vi "RT Main 9039.vi"() -> ()   [LabVIEW 2018]
doc: "This template is for the Queued Message Handler design pattern.\n\nThe Event Handling Loop generates messages based on user interface actions.\n\nThe Message Handling Loop processes messages generated by the Event Handling Loop, or by other messages. The messages are string values, so new messages can be added easily to the Message Cases case structure in the Message Handling Loop. Each message cluster can also provide an optional value for Message Data, which is a variant that can be converted to whatever message-specific data is required."
uses:
  controls/FPGA State.ctl
  controls/Fill Valves.ctl
  controls/VENT SYSTEM.ctl
  controls/LNG PUGE.ctl
  controls/LOX PURGE.ctl
  Globals/Global - All RT Loop Stop.vi
  Globals/Global - Configuration Options.vi
  COMET  Extra Programs/Globals/Global - Monitoring Variables.vi
  <vilib>/rvi/errors/niLvFpgaAdjustHostInterfaceError.vi
  Globals/Global - RT Stream Connections.vi
  <vilib>/FPGAPlugInAG/Dynamic/niLvFpga_Close_Dynamic.vi
  <vilib>/rvi/interface/nirviReadWriteControl/nirviReadWriteControl.xnode
  controls/FPGA VI Reference.ctl
  <vilib>/rvi/interface/nirviCloseFPGA/nirviCloseFPGA.xnode
  support/Message Queue/Message Queue.lvlib
  NiFpgaLv.dll
  <vilib>/rvi/interface/Simulation/niFpgaSimulationCallBeginRW.vi
  <vilib>/nisyscfg/nisyscfg.lvlib
panel:
  out "data 2":enum16{"Standard", "Grill", "ROFI"}(ring)
  out "MOD 2 error":bool
  out "Input Error":bool
  out "Watchdog Timed Out?":bool
  out "Current FPGA State":enum16{"Safe State", "Manual", "Control"}(ring)
  out "data":T1
  out "MOD 6 Error":bool
  out "LNG_BV":bool
  out "LOX_BV":bool
  out "dup error to report":errorcluster
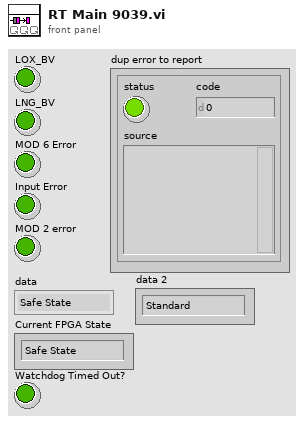
[diagram p1: front panel]
types:
  T1 = typedef "FPGA State.ctl" = enum16{"Safe State", "Manual", "Control"}
  T2 = typedef "Acquisition and Logging Configuration.ctl" = cluster{"Samples per Read 9237":i32, "Number of Reads to Save":i32, "Data File Name 9222_9039_EXP":string, "TDMS Properties 9222":T3[], "Number of Channels 9237_9049_MAIN":i32, "Trigger - RMS Value":dbl, "Trigger - Channel":i32, "Trigger - Time (Minute)":i32, "Data Rate 9237":T4, "Number of Channels 9222_9039_EXP":i32, "Samples per Read 9222":i32, "Data Rate 9222":i32, "Channel Names 9222_9039_EXP":string[], "TDMS Properties 9237":T3[], "Data File Name 9237_9049":string, "Excitation Voltage":T5, "Data File Name 9222_9049_MAIN":string, "Number of Channels 9222_9049_MAIN":i32, "Channel Names 9222_9049_MAIN":string[], "Data File Name 9237_9039":string, "Channel Names 9237_9039_EXP":string[], "Channel Names 9237_9049_MAIN":string[], "Number of Channels 9237_9039_EXP":i32}
  T3 = typedef "TDMS Properties.ctl" = cluster{"Name":string, "Value":string}
  T4 = typedef "nicrio_cRIO-9237_DataRatesRing.ctl" = u8
  T5 = typedef "nicrio_cRIO-9237_ExcitationVoltageRing.ctl" = u8
  T6 = typedef "EXPANSION FPGA VI Reference.ctl" = refnum<k20>
  T7 = typedef "FPGA VI Reference.ctl" = refnum<k20>
  T8 = typedef "Message Queue.lvlib/All Real-Time Message Queues Multi Queues.ctl" = cluster{"Message Handler":refnum<queue>, "Acquisition and Logging 9237":refnum<queue>, "Emergeny Stop for DCs":refnum<queue>, "LNG DC Commands":refnum<queue>, "LOX DC Commands":refnum<queue>, "Acquisition and Logging 9222":refnum<queue>, "Acquisition and Logging 9222_MAIN":refnum<queue>, "AUTO P&D":refnum<queue>, "Pressure Control":refnum<queue>}
  T9 = typedef "VENT SYSTEM.ctl" = cluster{"LNG_BFV":bool, "LOX_BFV":bool, "NGV_GV":bool}
  T10 = typedef "LNG PUGE.ctl" = cluster{"LNG_USP":bool, "LNG_DSP":bool}
  T11 = typedef "LOX PURGE.ctl" = cluster{"LOX_USP":bool, "LOX_DSP":bool}
  T12 = typedef "All FPGA Configuration Values.ctl" = cluster{"FPGA State":T1, "Manual Values":T13, "Fill Valves":T14, "LNG Purge System":T10, "LOX Purge System":T11, "DECOUPLERS":T15, "VENT SYSTEM":T9}
  T13 = typedef "Raw Values.ctl" = cluster{"LNG_VCV_POS":i16, " LOX_VCV_POS":i16, "LNG_VCV_CLOSE":bool, "LOX_VCV_CLOSE":bool, "LNG_BV_OPEN":bool, "LNG_BV_CLOSE":bool, "LOX_BV_OPEN":bool, "LOX_BV_CLOSE":bool, "LNG_BFV_OPEN":bool, "LNG_BFV_CLOSE":bool, "LOX_BFV_OPEN":bool, "LOX_BFV_CLOSE":bool}
  T14 = typedef "Fill Valves.ctl" = cluster{"LOX_BV":bool, "LNG_BV":bool, "LNG_VCV_CTL":sgl, "LOX_VCV_CTL":sgl}
  T15 = typedef "DECOUPLERS.ctl" = cluster{"LNG_DC":bool, "LOX_DC":bool, "NGV_DC":bool}
  T16 = cluster{"LOX_BV":bool, "LNG_BV":bool, "LNG_VCV_CTL":sgl, "LOX_VCV_CTL":sgl}
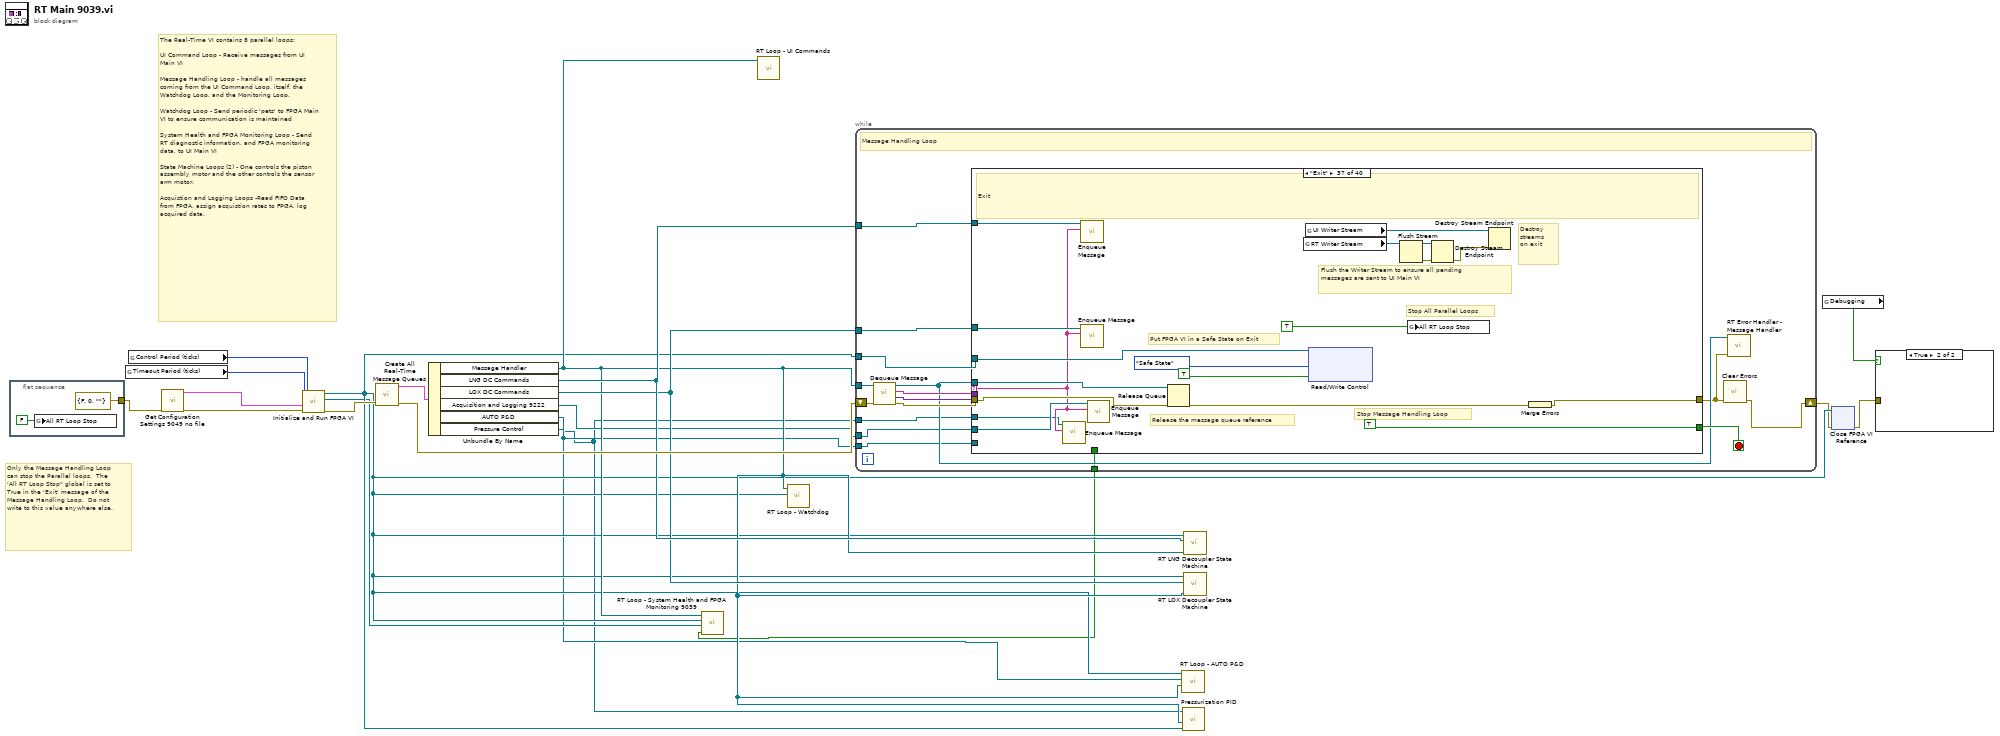
[diagram p0: block diagram]
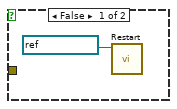
[diagram p2: hidden frame]
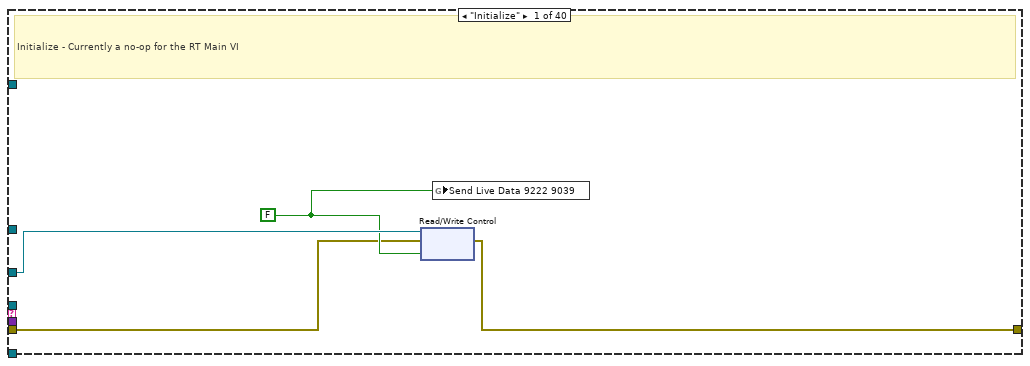
[diagram p3: hidden frame]
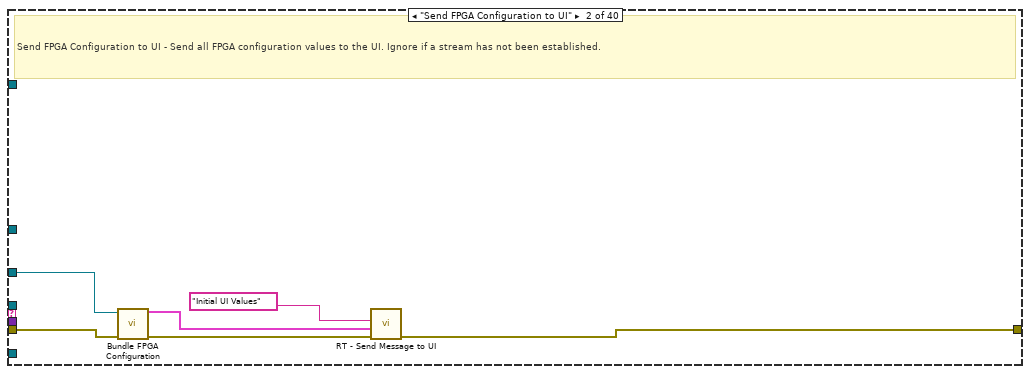
[diagram p4: hidden frame]
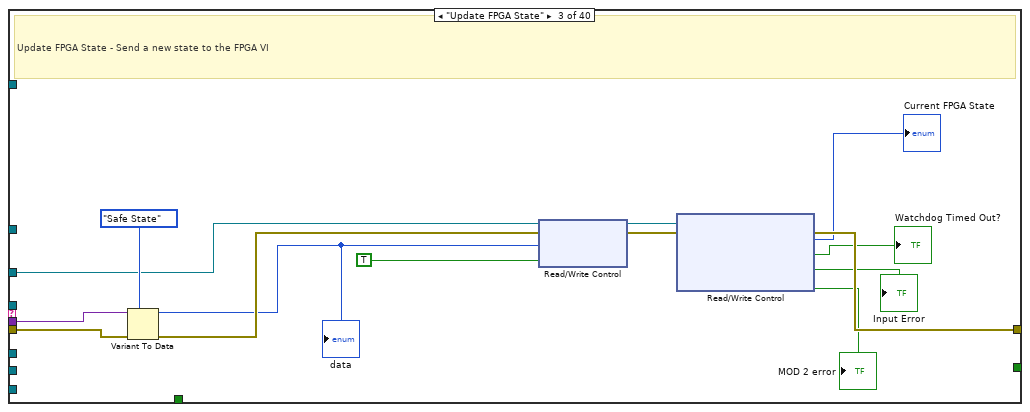
[diagram p5: hidden frame]
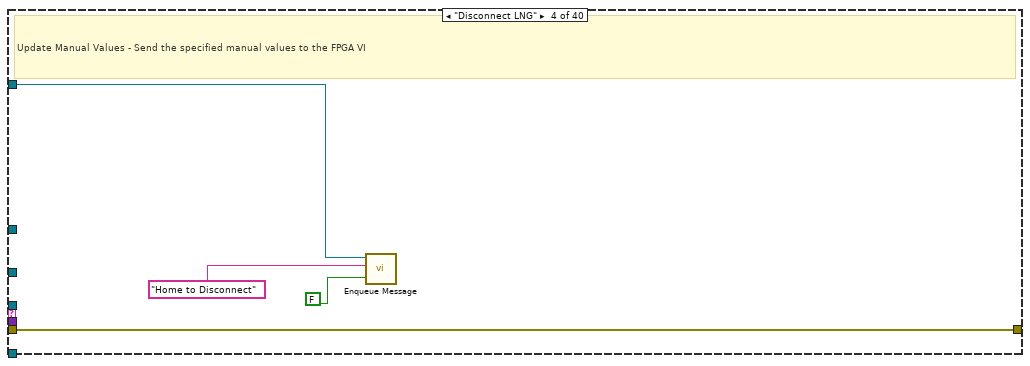
[diagram p6: hidden frame]
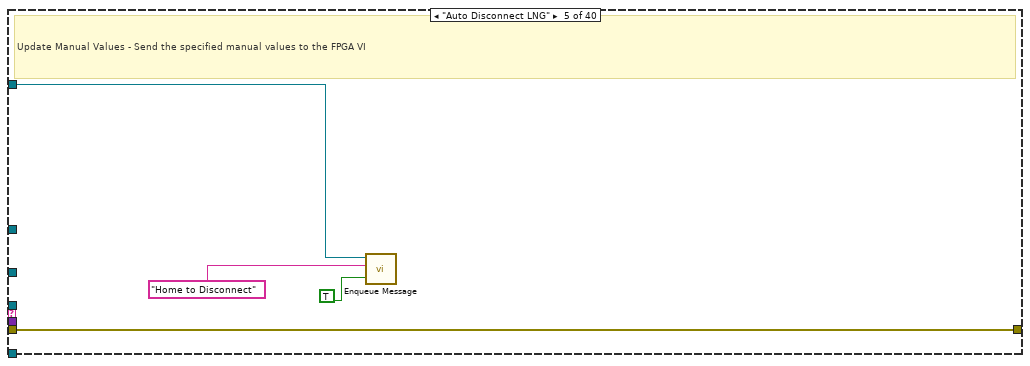
[diagram p7: hidden frame]
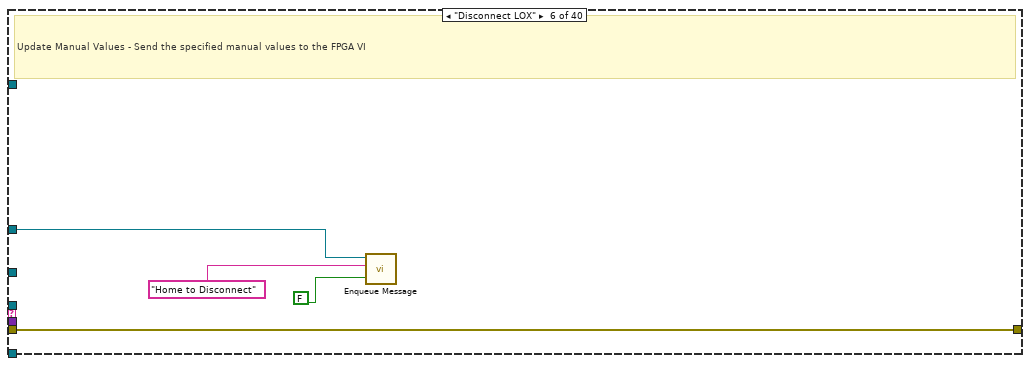
[diagram p8: hidden frame]
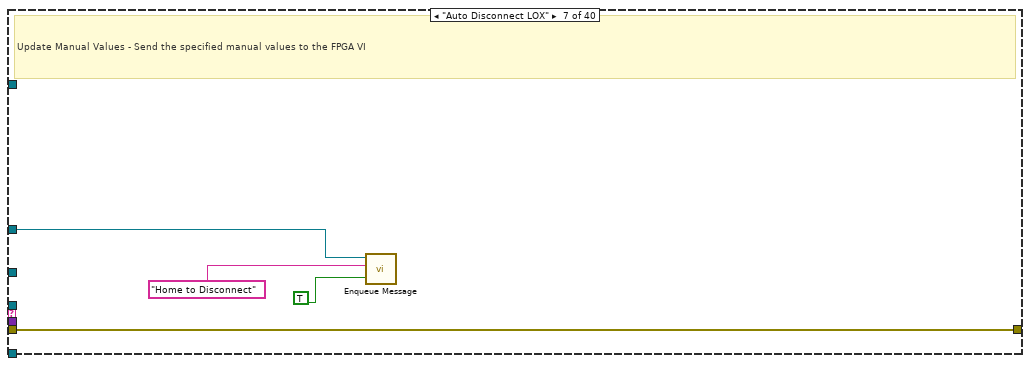
[diagram p9: hidden frame]
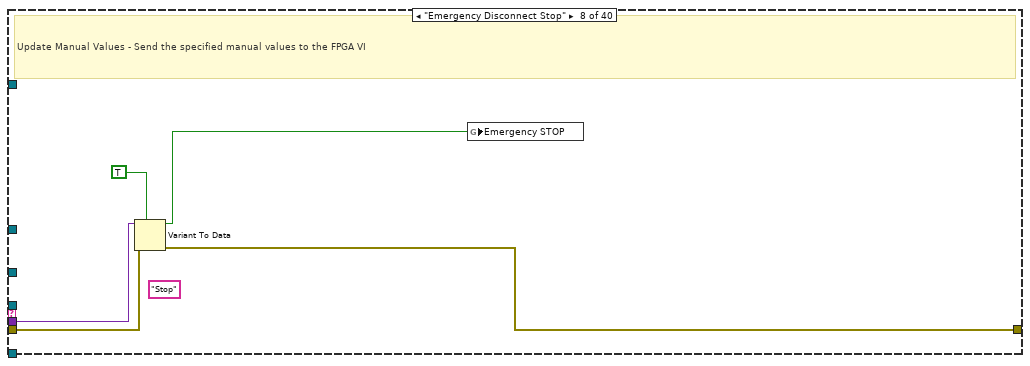
[diagram p10: hidden frame]
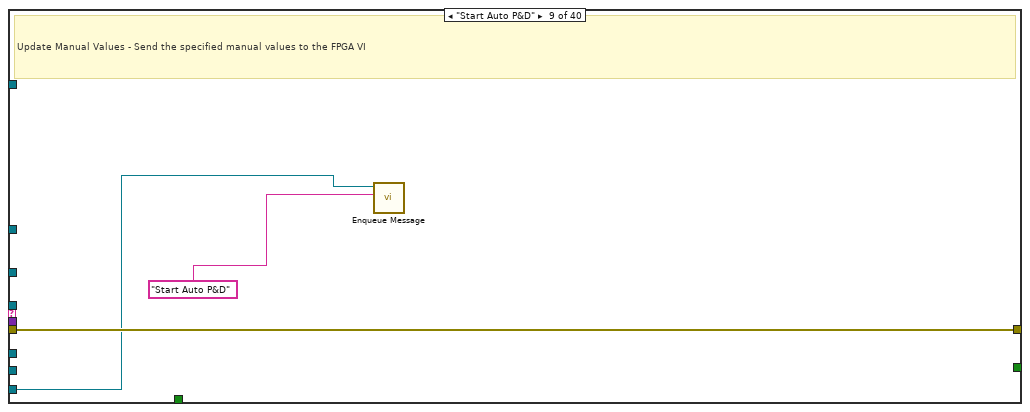
[diagram p11: hidden frame]
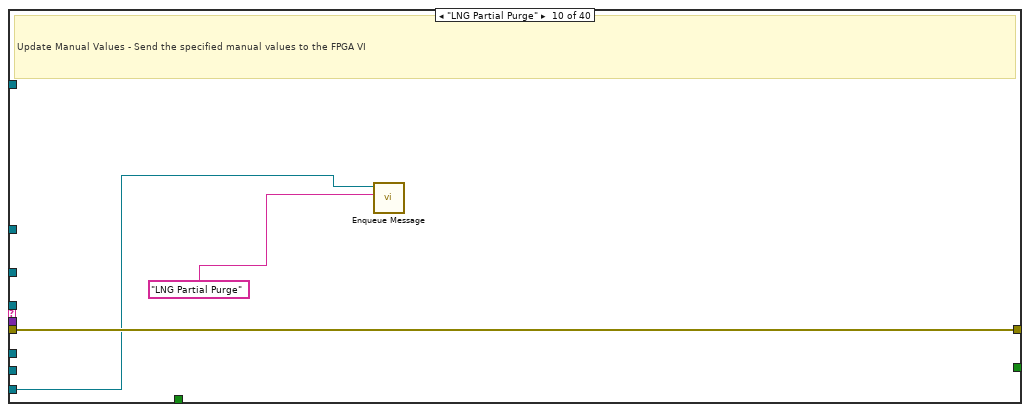
[diagram p12: hidden frame]
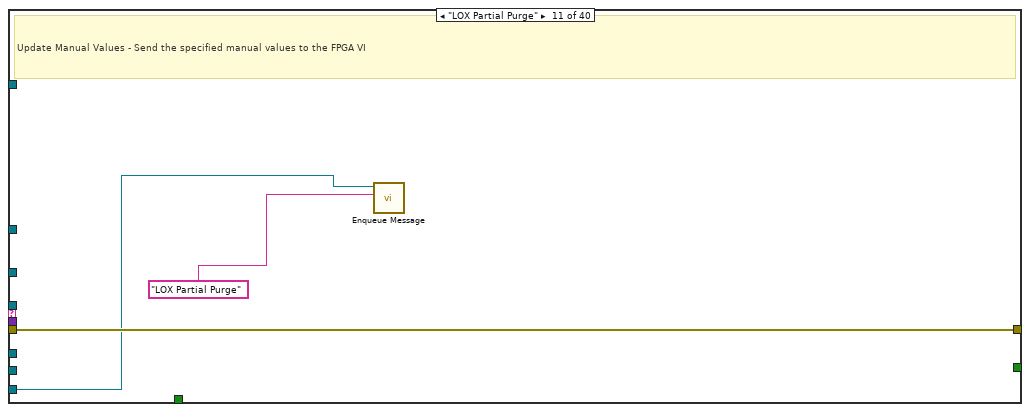
[diagram p13: hidden frame]
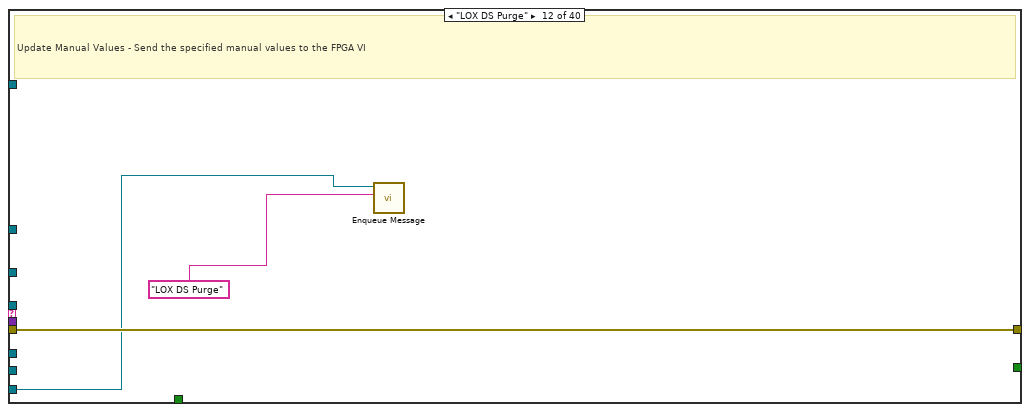
[diagram p14: hidden frame]
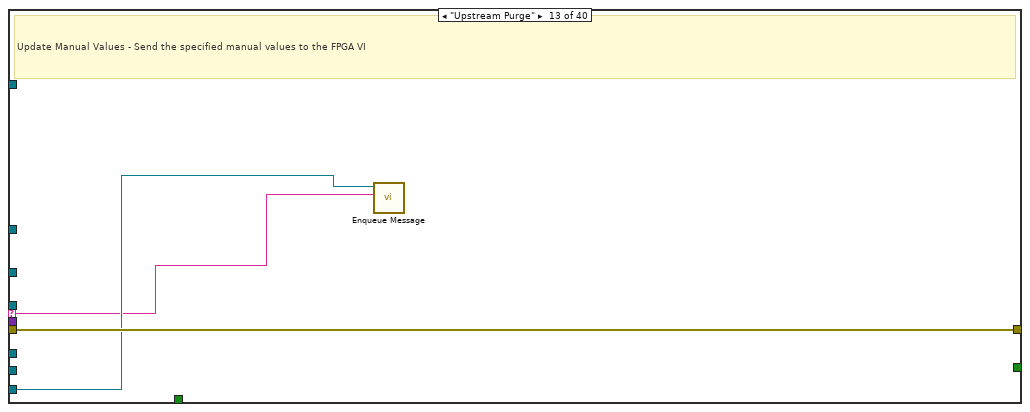
[diagram p15: hidden frame]
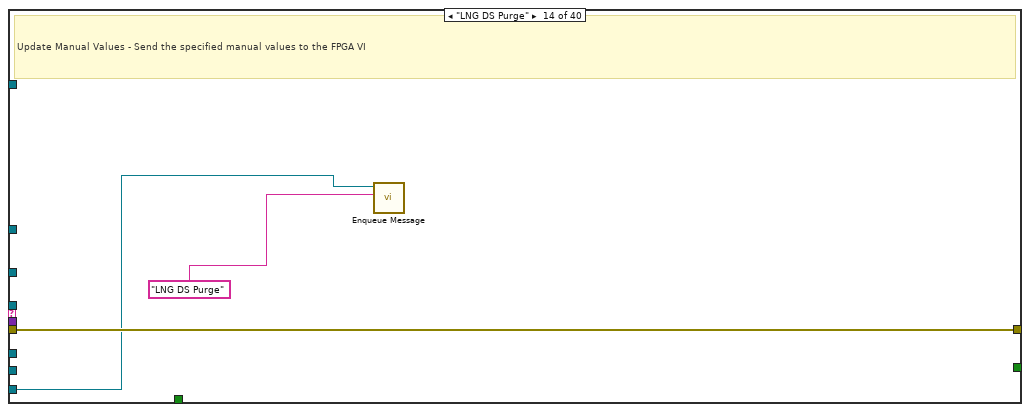
[diagram p16: hidden frame]
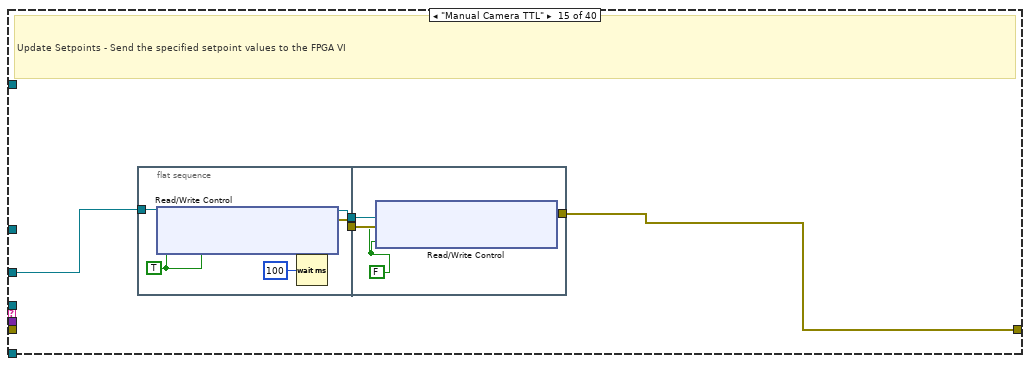
[diagram p17: hidden frame]
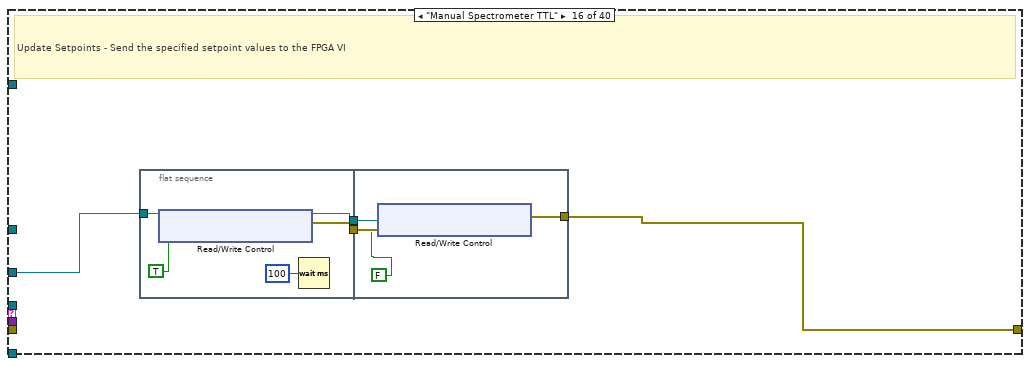
[diagram p18: hidden frame]
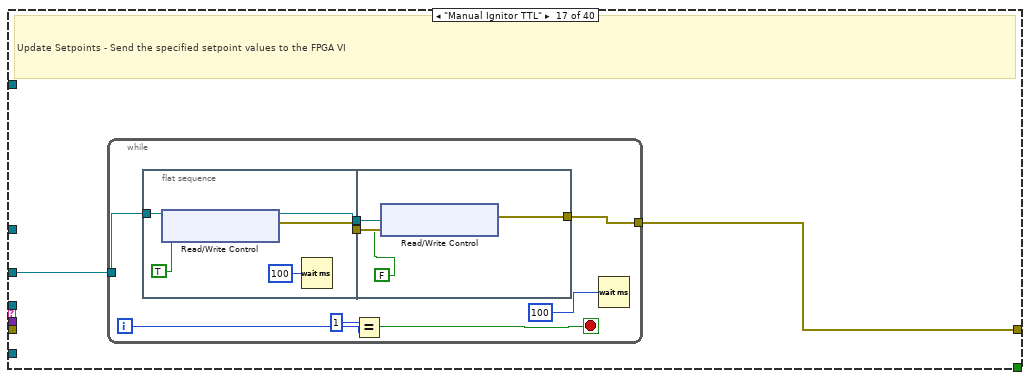
[diagram p19: hidden frame]
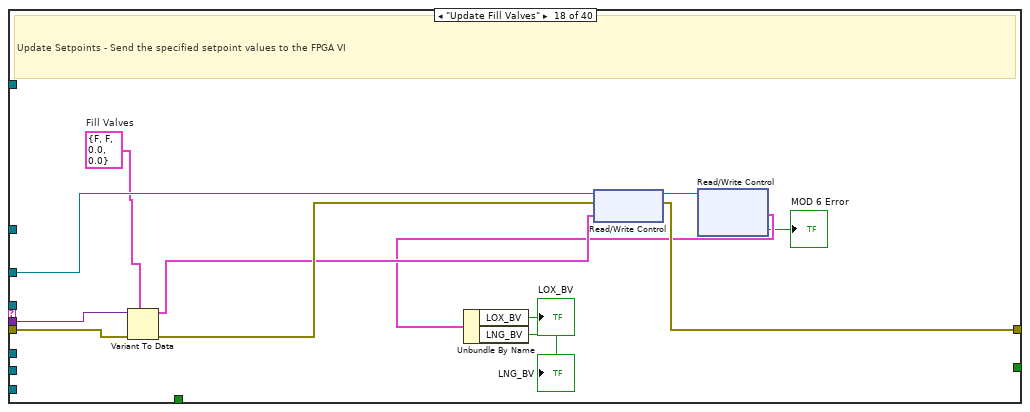
[diagram p20: hidden frame]
diagram:
  # "The Real-Time VI contains 8 parallel loops:\n\nUI Command Loop - Receive messages from UI Main VI\n\nMessage Handling Loop - handle all messages coming from the UI Command Loop, itself, the Watchdog Loop, and the Monitoring Loop.\n\nWatchdog Loop - Send periodic 'pets' to FPGA Main VI to ensure communication is maintained\n\nSystem Health and FPGA Monitoring Loop - Send RT diagnostic information, and FPGA monitoring data, to UI Main VI\n\nState Machine Loops (2) - One controls the piston assembly motor and the other controls the sensor arm motor.\n\nAcquistion and Logging Loops -Read FIFO Data from FPGA, assign acquistion rates to FPGA, log acquired data."
  # "Only the Message Handling Loop can stop the Parallel loops.  The 'All RT Loop Stop\" global is set to True in the 'Exit' message of the Message Handling Loop.  Do not write to this value anywhere else."
  n1 = flat-sequence {
    tunnel: [errorcluster {"status"=FALSE, "code"=0, "source"=""} ("error constant")] -> w10
    frame #0 {
      n2 = global write "Global - All RT Loop Stop.vi" "All RT Loop Stop"(FALSE) -> ()
    }
  }
  n3 = global read "Global - Configuration Options.vi" "Timeout Period (ticks)"() -> (w20:u64)
  n4 = global read "Global - Configuration Options.vi" "Control Period (ticks)"() -> (w19:u32)
  n5 = call "Get Configuration Settings 9049 no file.vi"("error in (no error)"=w10) -> ("error out"=w11:errorcluster, "Acquisition and Logging Configuration"=w12:T2)  [unwired: 9 in]
  n6 = call "Initialize and Run FPGA VI.vi"("error in (no error)"=w11, "Acquisition and Logging Configuration"=w12, "Timeout Period (ticks)"=w20, "Control Period (ticks)"=w19) -> ("error out"=w17:errorcluster, "EXPANSION FPGA VI Reference Out"=w4:T6, "FPGA VI Reference"=w8:T7)  [unwired: 4 in, 1 out]
  n7 = call "Create All Real-Time Message Queues.vi"("error in (no error)"=w17) -> ("error out"=w15:errorcluster, "Message Queues out"=w16:T8)  [unwired: 9 in]
  n8 = Unbundle By Name(w16) -> ("Message Handler"=w9:refnum<queue>, "LNG DC Commands"=w14:refnum<queue>, "LOX DC Commands"=w13:refnum<queue>, "Acquisition and Logging 9222"=w3:refnum<queue>, "AUTO P&D"=w2:refnum<queue>, "Pressure Control"=w1:refnum<queue>)
  n9 = call "RT Loop - UI Commands.vi"("Message Queue"=w9) -> ()  [unwired: 11 in]
  n10 = call "RT Loop - Watchdog.vi"("FPGA VI Reference"=w8, "Message Queue"=w9) -> ()  [unwired: 10 in]
  n11 = while {
    tunnel: w9 -> [w33]
    shift-right: [w24] -> w6
    shift-left: w15 -> [w37]
    tunnel: w8 -> [w32]
    tunnel: w13 -> [w29]
    tunnel: w14 -> [w28]
    tunnel: w3 -> [w27]
    tunnel: w2 -> [w26]
    tunnel: w1 -> [w25]
    tunnel: [w23] -> w5
    stop <- w38 stop-if-true
    # "Message Handling Loop"
    n12 = call "Dequeue Message.vi"("error in (no error)"=w37, "Message Queue"=w33) -> ("error out"=w36:errorcluster, "Message Data"=w34:variant, "Message"=w35:string, "dup Message Queue"=w31:refnum<queue>)  [unwired: 6 in]
    n13 = case "Message Cases" shown="\"Exit\"" w35 {
      selector: w35 -> [_ _ _ _ _ _ _ _ _ _ _ _ w95 _ _ _ _ _ _ _ _ _ _ _ _ w217 w221 _ _ w233 _ w244 w248 _ w262 w278 w306 _ _ w337]
      tunnel: w31 -> [_ _ _ _ _ _ _ _ _ _ _ _ _ _ _ _ _ _ _ _ _ _ _ _ _ _ _ _ _ _ _ _ _ _ _ w272 w323 _ _ _]
      tunnel: w36 -> [w40 w48 w61 w65 w69 w72 w76 w79 w85 w88 w91 w94 w97 w100 _ _ _ w157 w160 w169 w172 w181 w188 w195 w202 w215 w219 w225 w230 w238 w242 w246 w250 w261 w266 w276 w319 w325 w330 _]
      tunnel: [w39 w43 w58 w65 w69 w72 w76 w78 w85 w88 w91 w94 w97 w100 w101 w114 w127 w152 w159 w165 w171 w177 w183 w191 w198 w218 w222 w224 w229 w238 w241 w245 w249 w252 w263 w277 w320 w324 w329 w335] -> w30
      tunnel: [_ _ _ _ _ _ _ _ _ _ _ _ _ _ _ _ _ _ _ _ _ _ _ _ _ _ _ _ _ _ _ _ _ _ _ _ TRUE _ _ _] -> w38
      tunnel: w34 -> [_ _ w60 _ _ _ _ w82 _ _ _ _ _ _ _ _ _ w156 w158 w168 w174 w180 w187 w194 w201 w213 _ w223 w228 _ w240 _ _ w260 w265 w275 _ _ _ _]
      tunnel: w32 -> [w42 w47 w56 _ _ _ _ _ _ _ _ _ _ _ w102 w115 w128 w155 _ w167 _ w179 w186 w193 w200 w211 _ _ _ _ _ _ _ _ _ _ w315 _ _ _]
      tunnel: w29 -> [_ _ _ _ _ w73 w77 _ _ _ _ _ _ _ _ _ _ _ _ _ _ _ _ _ _ _ _ _ _ _ _ _ _ _ _ _ w307 _ _ _]
      tunnel: w28 -> [_ _ _ w63 w67 _ _ _ _ _ _ _ _ _ _ _ _ _ _ _ _ _ _ _ _ _ _ _ _ _ _ _ _ _ _ _ w308 _ _ _]
      tunnel: w27 -> [_ _ _ _ _ _ _ _ _ _ _ _ _ _ _ _ _ _ _ _ _ _ _ _ _ w216 w220 _ _ _ _ _ _ _ _ _ w309 _ _ _]
      tunnel: w26 -> [_ _ _ _ _ _ _ _ w83 w86 w89 w92 w96 w98 _ _ _ _ _ _ _ _ _ _ _ _ _ _ _ _ _ _ _ _ _ _ _ _ w328 _]
      tunnel: w25 -> [_ _ _ _ _ _ _ _ _ _ _ _ _ _ _ _ _ _ w162 _ _ _ _ _ _ _ _ _ _ _ _ _ _ _ _ _ w305 _ _ _]
      tunnel: [_ _ _ _ _ _ _ _ _ _ _ _ _ _ _ _ _ _ _ _ w170 _ _ _ _ _ _ _ _ _ _ _ _ _ _ _ _ _ _ _] -> w23
      frame "Initialize" {
        w41 = FALSE
        # "Initialize - Currently a no-op for the RT Main VI"
        n14 = xnode "Read/Write Control"("FPGA VI Reference In"=w42, "error in"=w40, "FIRE"=w41) -> ("error out"=w39:errorcluster)  [unwired: 1 out]
        n15 = global write "Global - Monitoring Variables.vi" "Send Live Data 9222 9039"(w41) -> ()
      }
      frame "Send FPGA Configuration to UI" {
        # "Send FPGA Configuration to UI - Send all FPGA configuration values to the UI. Ignore if a stream has not been established."
        n16 = call "Bundle FPGA Configuration.vi"("error in (no error)"=w48, "FPGA Interface"=w47) -> ("error out"=w46:errorcluster, "All FPGA Configuration Values"=w45:T12)  [unwired: 8 in]
        n17 = call "RT - Send Message to UI.vi"("error in (no error)"=w46, "Message Data"=w45, "Message"="Initial UI Values") -> ("error out"=w43:errorcluster)  [unwired: 8 in]
      }
      frame "Update FPGA State" {
        # "Update FPGA State - Send a new state to the FPGA VI"
        n18 = Variant To Data(error in=w61, type=FPGA_State."Safe State" ("FPGA State"), Variant=w60) -> (data=w55:T1, error out=w57:errorcluster)
        "data" <- w55
        n19 = xnode "Read/Write Control"("FPGA VI Reference In"=w56, "error in"=w57, "New State"=w55, "Change State"=TRUE) -> ("FPGA VI Reference Out"=w53:T7, "error out"=w58:errorcluster)
        n20 = xnode "Read/Write Control"("FPGA VI Reference In"=w53) -> ("Current FPGA State"=→"Current FPGA State":enum16{"Safe State", "Manual", "Control"}, "Watchdog Timed Out?"=→"Watchdog Timed Out?":bool, "Input Error"=→"Input Error":bool, "9265 Error"=→"MOD 2 error":bool)  [unwired: 1 in, 2 out]
      }
      frame "Disconnect LNG" {
        # "Update Manual Values - Send the specified manual values to the FPGA VI"
        n21 = call "Enqueue Message.vi"("Message Data"=FALSE, "Message"="Home to Disconnect", "Message Queue"=w63) -> ()  [unwired: 7 in, 2 out]
      }
      frame "Auto Disconnect LNG" {
        # "Update Manual Values - Send the specified manual values to the FPGA VI"
        n22 = call "Enqueue Message.vi"("Message Data"=TRUE, "Message"="Home to Disconnect", "Message Queue"=w67) -> ()  [unwired: 7 in, 2 out]
      }
      frame "Disconnect LOX" {
        # "Update Manual Values - Send the specified manual values to the FPGA VI"
        n23 = call "Enqueue Message.vi"("Message Data"=FALSE, "Message"="Home to Disconnect", "Message Queue"=w73) -> ()  [unwired: 7 in, 2 out]
      }
      frame "Auto Disconnect LOX" {
        # "Update Manual Values - Send the specified manual values to the FPGA VI"
        n24 = call "Enqueue Message.vi"("Message Data"=TRUE, "Message"="Home to Disconnect", "Message Queue"=w77) -> ()  [unwired: 7 in, 2 out]
      }
      frame "Emergency Disconnect Stop" {
        (unwired) "Stop" ("Message")
        # "Update Manual Values - Send the specified manual values to the FPGA VI"
        n25 = Variant To Data(error in=w79, type=TRUE ("Priority Message? (F)"), Variant=w82) -> (data=w80:bool, error out=w78:errorcluster)
        n26 = global write "Global - Monitoring Variables.vi" "Emergency STOP"(w80) -> ()
      }
      frame "Start Auto P&D" {
        # "Update Manual Values - Send the specified manual values to the FPGA VI"
        n27 = call "Enqueue Message.vi"("Message"="Start Auto P&D", "Message Queue"=w83) -> ()  [unwired: 8 in, 2 out]
      }
      frame "LNG Partial Purge" {
        # "Update Manual Values - Send the specified manual values to the FPGA VI"
        n28 = call "Enqueue Message.vi"("Message"="LNG Partial Purge", "Message Queue"=w86) -> ()  [unwired: 8 in, 2 out]
      }
      frame "LOX Partial Purge" {
        # "Update Manual Values - Send the specified manual values to the FPGA VI"
        n29 = call "Enqueue Message.vi"("Message"="LOX Partial Purge", "Message Queue"=w89) -> ()  [unwired: 8 in, 2 out]
      }
      frame "LOX DS Purge" {
        # "Update Manual Values - Send the specified manual values to the FPGA VI"
        n30 = call "Enqueue Message.vi"("Message"="LOX DS Purge", "Message Queue"=w92) -> ()  [unwired: 8 in, 2 out]
      }
      frame "Upstream Purge" {
        # "Update Manual Values - Send the specified manual values to the FPGA VI"
        n31 = call "Enqueue Message.vi"("Message"=w95, "Message Queue"=w96) -> ()  [unwired: 8 in, 2 out]
      }
      frame "LNG DS Purge" {
        # "Update Manual Values - Send the specified manual values to the FPGA VI"
        n32 = call "Enqueue Message.vi"("Message"="LNG DS Purge", "Message Queue"=w98) -> ()  [unwired: 8 in, 2 out]
      }
      frame "Manual Camera TTL" {
        # "Update Setpoints - Send the specified setpoint values to the FPGA VI"
        n33 = flat-sequence {
          tunnel: [w109] -> w104
          tunnel: [w108] -> w103
          tunnel: w102 -> [w105]
          tunnel: w104 -> [w113]
          tunnel: w103 -> [w112]
          tunnel: [w110] -> w101
          frame #0 {
            w106 = TRUE ("Manual Camera TTL Secondary")
            n34 = xnode "Read/Write Control"("FPGA VI Reference In"=w105, "Manual Camera TTL"=w106, "Manual Camera TTL Secondary"=w106) -> ("FPGA VI Reference Out"=w108:T7, "error out"=w109:errorcluster)  [unwired: 1 in]
            n35 = Wait (ms)(milliseconds to wait=u32 100) -> ()  [unwired: 1 out]
          }
          frame #1 {
            w111 = FALSE ("Manual Camera TTL Secondary")
            n36 = xnode "Read/Write Control"("FPGA VI Reference In"=w112, "error in"=w113, "Manual Camera TTL"=w111, "Manual Camera TTL Secondary"=w111) -> ("error out"=w110:errorcluster)  [unwired: 1 out]
          }
        }
      }
      frame "Manual Spectrometer TTL" {
        # "Update Setpoints - Send the specified setpoint values to the FPGA VI"
        n37 = flat-sequence {
          tunnel: [w122] -> w117
          tunnel: [w121] -> w116
          tunnel: w115 -> [w118]
          tunnel: w117 -> [w126]
          tunnel: w116 -> [w125]
          tunnel: [w123] -> w114
          frame #0 {
            n38 = xnode "Read/Write Control"("FPGA VI Reference In"=w118, "Manual Spectrometer TTL"=TRUE ("Manual Camera TTL Secondary")) -> ("FPGA VI Reference Out"=w121:T7, "error out"=w122:errorcluster)  [unwired: 1 in]
            n39 = Wait (ms)(milliseconds to wait=u32 100) -> ()  [unwired: 1 out]
          }
          frame #1 {
            n40 = xnode "Read/Write Control"("FPGA VI Reference In"=w125, "error in"=w126, "Manual Spectrometer TTL"=FALSE ("Manual Camera TTL Secondary")) -> ("error out"=w123:errorcluster)  [unwired: 1 out]
          }
        }
      }
      frame "Manual Ignitor TTL" {
        # "Update Setpoints - Send the specified setpoint values to the FPGA VI"
        n41 = while {
          tunnel: w128 -> [w134]
          tunnel: [w133] -> w127
          i -> [w132]
          stop <- w129 stop-if-true
          n42 = flat-sequence {
            tunnel: [w141] -> w136
            tunnel: [w140] -> w135
            tunnel: w134 -> [w137]
            tunnel: w136 -> [w145]
            tunnel: w135 -> [w144]
            tunnel: [w142] -> w133
            frame #0 {
              n43 = xnode "Read/Write Control"("FPGA VI Reference In"=w137, "Manual Ignitor TTL"=TRUE ("Manual Camera TTL Secondary")) -> ("FPGA VI Reference Out"=w140:T7, "error out"=w141:errorcluster)  [unwired: 1 in]
              n44 = Wait (ms)(milliseconds to wait=u32 100) -> ()  [unwired: 1 out]
            }
            frame #1 {
              n45 = xnode "Read/Write Control"("FPGA VI Reference In"=w144, "error in"=w145, "Manual Ignitor TTL"=FALSE ("Manual Camera TTL Secondary")) -> ("error out"=w142:errorcluster)  [unwired: 1 out]
            }
          }
          n46 = Equal?(x=1, y=w132) -> (x = y?=w129:bool)
          n47 = Wait (ms)(milliseconds to wait=u32 100) -> ()  [unwired: 1 out]
        }
      }
      frame "Update Fill Valves" {
        w154 = T14 {"LOX_BV"=FALSE, "LNG_BV"=FALSE, "LNG_VCV_CTL"=0.0, "LOX_VCV_CTL"=0.0}  # Fill Valves
        # "Update Setpoints - Send the specified setpoint values to the FPGA VI"
        n48 = Variant To Data(error in=w157, type=w154, Variant=w156) -> (data=w151:T14, error out=w153:errorcluster)
        n49 = xnode "Read/Write Control"("FPGA VI Reference In"=w155, "error in"=w153, "Fill Valves"=w151) -> ("FPGA VI Reference Out"=w148:T7, "error out"=w152:errorcluster)
        n50 = xnode "Read/Write Control"("FPGA VI Reference In"=w148) -> ("Fill Valves"=w147:T16, "9264 Error"=→"MOD 6 Error":bool)  [unwired: 1 in, 2 out]
        n51 = Unbundle By Name(w147) -> ("LOX_BV"=→"LOX_BV":bool, "LNG_BV"=→"LNG_BV":bool)
      }
      frame "Update Tank Pressure" {
        # "Update Setpoints - Send the specified setpoint values to the FPGA VI"
        n52 = call "Enqueue Message.vi"("error in (no error)"=w160, "Message Data"=w158, "Message"="Tank Pressure", "Message Queue"=w162) -> ("error out"=w159:errorcluster)  [unwired: 6 in, 1 out]
      }
      frame "Update Vent System" {
        # "Update Setpoints - Send the specified setpoint values to the FPGA VI"
        n53 = Variant To Data(error in=w169, type=T9 {"LNG_BFV"=FALSE, "LOX_BFV"=FALSE, "NGV_GV"=FALSE} ("VENT SYSTEM"), Variant=w168) -> (data=w163:T9, error out=w166:errorcluster)
        n54 = xnode "Read/Write Control"("FPGA VI Reference In"=w167, "error in"=w166, "VENT SYSTEM"=w163) -> ("error out"=w165:errorcluster)  [unwired: 1 out]
      }
      frame "Expansion Chassis" {
        n55 = Variant To Data(error in=w172, type=TRUE, Variant=w174) -> (data=w170:bool, error out=w171:errorcluster)
      }
      frame "Update NG_PVC_BV" {
        # "Update Setpoints - Send the specified setpoint values to the FPGA VI"
        n56 = Variant To Data(error in=w181, type=TRUE, Variant=w180) -> (data=w176:bool, error out=w178:errorcluster)
        n57 = xnode "Read/Write Control"("FPGA VI Reference In"=w179, "error in"=w178, "PVC Vent"=w176) -> ("error out"=w177:errorcluster)  [unwired: 1 out]
      }
      frame "Update LNG Purge System" {
        # "Update Setpoints - Send the specified setpoint values to the FPGA VI"
        n58 = Variant To Data(error in=w188, type=T10 {"LNG_USP"=FALSE, "LNG_DSP"=FALSE} ("Purge System"), Variant=w187) -> (data=w185:T10, error out=w184:errorcluster)
        n59 = xnode "Read/Write Control"("FPGA VI Reference In"=w186, "error in"=w184, "LNG PURGE"=w185) -> ("error out"=w183:errorcluster)  [unwired: 1 out]
      }
      frame "Update LOX Purge System" {
        # "Update Setpoints - Send the specified setpoint values to the FPGA VI"
        n60 = Variant To Data(error in=w195, type=T11 {"LOX_USP"=FALSE, "LOX_DSP"=FALSE} ("Purge System"), Variant=w194) -> (data=w190:T11, error out=w192:errorcluster)
        n61 = xnode "Read/Write Control"("FPGA VI Reference In"=w193, "error in"=w192, "LOX PURGE"=w190) -> ("error out"=w191:errorcluster)  [unwired: 1 out]
      }
      frame "Arm" {
        # "Update Setpoints - Send the specified setpoint values to the FPGA VI"
        n62 = Variant To Data(error in=w202, type=TRUE, Variant=w201) -> (data=w197:bool, error out=w199:errorcluster)
        n63 = xnode "Read/Write Control"("FPGA VI Reference In"=w200, "error in"=w199, "Arm"=w197) -> ("error out"=w198:errorcluster)  [unwired: 1 out]
      }
      frame "Force Trigger" {
        w209 = enum16{"Standard", "Grill", "ROFI"}."Standard" ("Mode")
        # "Force Trigger - Send a message to the Acquisition and Logging loop to trigger a manual log file.\n\nGet Logging Status - Figure out if the logging loop is functioning normally, or if it is in a safe state.\n\nStart Logging - Move the Acquisition and Logging Loop out of safe state, if it's not already."
        n64 = xnode "Read/Write Control"("FPGA VI Reference In"=w211, "TTL State"=enum16{"AUTO", "MANUAL", "OFF"}."AUTO", "HP Duration (ms)"=u32 10000 ("Spark Duration (ms)"), "Photo Delay (ms)"=u32 500 ("Spark Duration (ms)"), "2nd IGN Delay (ms) 2"=u32 3000 ("2nd IGN Delay (ms)")) -> ("FPGA VI Reference Out"=w208:T7)  [unwired: 1 in, 1 out]
        n65 = call "Enqueue Message.vi"("Message"=w217, "Message Queue"=w216) -> ("error out"=w212:errorcluster)  [unwired: 8 in, 1 out]
        n66 = Variant To Data(error in=w215, type=w209, Variant=w213) -> (data=→"data 2":enum16{"Standard", "Grill", "ROFI"}, error out=w214:errorcluster)
        n67 = xnode "Read/Write Control"("FPGA VI Reference In"=w208, "FIRE"=TRUE) -> ()  [unwired: 1 in, 2 out]
        n68 = global write "Global - Monitoring Variables.vi" "Fire Mode"(w209) -> ()
        n69 = Merge Errors(w212, w214) -> (w218:errorcluster)
      }
      frame "Get Logging Status 9039", "Start Logging" {
        # "Force Trigger - Send a message to the Acquisition and Logging loop to trigger a manual log file.\n\nGet Logging Status - Figure out if the logging loop is functioning normally, or if it is in a safe state.\n\nStart Logging - Move the Acquisition and Logging Loop out of safe state, if it's not already."
        n70 = call "Enqueue Message.vi"("Message"=w221, "Message Queue"=w220) -> ()  [unwired: 8 in, 2 out]
        n71 = Merge Errors(w219) -> (w222:errorcluster)
      }
      frame "Live Channel Change 9222 9039" {
        # "Live Channel Change - This message came from the UI Main VI.  Change the global that stores which channel's data is being streamed to the UI."
        n72 = Variant To Data(error in=w225, type=u32 0, Variant=w223) -> (data=w227:u32, error out=w224:errorcluster)
        n73 = global write "Global - Monitoring Variables.vi" "Live Data Channel 9222 9039"(w227) -> ()
      }
      frame "Live Channel Change 9237 9039" {
        # "Live Channel Change - This message came from the UI Main VI.  Change the global that stores which channel's data is being streamed to the UI."
        n74 = Variant To Data(error in=w230, type=u32 0, Variant=w228) -> (data=w232:u32, error out=w229:errorcluster)
        n75 = global write "Global - Monitoring Variables.vi" "Live Data Channel 9237 9039"(w232) -> ()
      }
      frame "Acquire Live Data 9222 9039", "Acquire Live Data 9237 9039", "Stop Live Data 9039" {
        n76 = Equal?(x="Acquire Live Data 9222 9039", y=w233) -> (x = y?=w236:bool)
        n77 = Equal?(x="Acquire Live Data 9237 9039", y=w233) -> (x = y?=w235:bool)
        n78 = global write "Global - Monitoring Variables.vi" "Send Live Data 9222 9039"(w236) -> ()
        n79 = global write "Global - Monitoring Variables.vi" "Send Live Data 9237 9039"(w235) -> ()
      }
      frame "Send Mode Change to UI" {
        # "Send Mode Change to UI - Let the UI Main VI know that the mode of the FPGA Main VI has changed."
        n80 = call "RT - Send Message to UI.vi"("error in (no error)"=w242, "Message Data"=w240, "Message"="Update Display Mode") -> ("error out"=w241:errorcluster)  [unwired: 8 in]
      }
      frame "Auto P&D No Start", "LNG DC Complete", "LOX DC Complete", "Request UI to DC LNG", "Request UI to DC LOX", "System Lockup Complete" {
        # "Send Mode Change to UI - Let the UI Main VI know that the mode of the FPGA Main VI has changed."
        n81 = call "RT - Send Message to UI.vi"("error in (no error)"=w246, "Message Data"=TRUE, "Message"=w244) -> ("error out"=w245:errorcluster)  [unwired: 8 in]
      }
      frame "Manual LNG DC Complete", "Manual LOX DC Complete", "Manual NGV DC Complete" {
        # "Send Mode Change to UI - Let the UI Main VI know that the mode of the FPGA Main VI has changed."
        n82 = call "RT - Send Message to UI.vi"("error in (no error)"=w250, "Message Data"=TRUE, "Message"=w248) -> ("error out"=w249:errorcluster)  [unwired: 8 in]
      }
      frame "Log Error" {
        # "Log Error - Log the error, along with a timestamp, to the RT log file."
        n83 = Variant To Data(error in=w261, type=errorcluster {"status"=FALSE, "code"=0, "source"=""} ("error constant"), Variant=w260) -> (data=w255:errorcluster, error out=w258:errorcluster)
        n84 = Unbundle By Name(w255) -> ("code"=w254:i32, "source"=w253:string)
        n85 = Format Date/Time String() -> (date/time string=w256:string)  [unwired: 3 in]
        n86 = Format Into String(format string="\n%s: RT Error %d - %s", w256, w254, w253) -> (resulting string=w251:string)  [unwired: 2 in, 1 out]
        n87 = call "Write to RT Error Log.vi"("error in (no error)"=w258, "Log Entry"=w251) -> ("error out"=w252:errorcluster)  [unwired: 9 in]
      }
      frame "Send Error to UI", "Send Logging Status 9222 9039", "Send Logging Status 9237 9039", "Send Path to UI 9222 9039", "Send Path to UI 9237 9039" {
        # "Send Error to UI - Send the error message to the UI. Ignore if a stream has not been established."
        n88 = case shown="\"False\", Default" w262 {
          selector: w262 -> [w267 _]
          tunnel: [w267 "RT Error" ("Message")] -> w264
          frame "False", Default {
          }
          frame "Send Error To UI" {
          }
        }
        n89 = call "RT - Send Message to UI.vi"("error in (no error)"=w266, "Message Data"=w265, "Message"=w264) -> ("error out"=w263:errorcluster)  [unwired: 8 in]
      }
      frame "Critical Error", "Log-Only Error", "Non-Critical Error" {
        # "Note that the \"Should Log Error.vi\" checks to see if a duplicate error has occurred \nwithin a specified interval and if so, it is not logged."
        # "Error - Log the error, and send it to the UI.  If it's a critical error, shut down this VI with an 'Exit' message. If it's non-critical, put the FPGA in a Safe State. For anything else, no further action."
        n90 = Variant To Data(error in=w276, type=errorcluster {"status"=FALSE, "code"=0, "source"=""} ("error out"), Variant=w275) -> (data=w269:errorcluster, error out=w273:errorcluster)
        n91 = call "Should Log Error.vi"("error to report"=w269) -> ("Should Log Error?"=w271:bool, "dup error to report"=w270:errorcluster)  [unwired: 9 in]
        n92 = case shown="True" w271 {
          tunnel: [w282 w289] -> w280
          tunnel: [w281 w288] -> w279
          tunnel: w272 -> [w281 w287]
          tunnel: w273 -> [w282 w284]
          tunnel: w270 -> [_ w283]
          frame False {
          }
          frame True {
            n93 = call "Enqueue Message.vi"("error in (no error)"=w284, "Message Data"=w283, "Message"="Log Error", "Message Queue"=w287) -> ("error out"=w285:errorcluster, "dup Message Queue"=w286:refnum<queue>)  [unwired: 6 in]
            n94 = call "Enqueue Message.vi"("error in (no error)"=w285, "Message Data"=w283, "Message"="Send Error to UI", "Message Queue"=w286) -> ("error out"=w289:errorcluster, "dup Message Queue"=w288:refnum<queue>)  [unwired: 6 in]
            "dup error to report" <- w283
          }
        }
        n95 = case shown="\"Critical Error\"" w278 {
          tunnel: w280 -> [w295 w303 w304]
          tunnel: w279 -> [w293 w302 _]
          tunnel: [w294 w299 w304] -> w277
          frame "Critical Error" {
            n96 = call "Enqueue Message.vi"("error in (no error)"=w295, "Message"="Exit", "Message Queue"=w293) -> ("error out"=w294:errorcluster)  [unwired: 7 in, 1 out]
          }
          frame "Non-Critical Error" {
            w296 = FPGA_State."Safe State" ("FPGA State")
            n97 = call "Enqueue Message.vi"("error in (no error)"=w303, "Message Data"=w296, "Message"="Update FPGA State", "Message Queue"=w302) -> ("error out"=w300:errorcluster, "dup Message Queue"=w297:refnum<queue>)  [unwired: 6 in]
            n98 = call "Enqueue Message.vi"("error in (no error)"=w300, "Message Data"=w296, "Message"="Send Mode Change to UI", "Message Queue"=w297) -> ("error out"=w299:errorcluster)  [unwired: 6 in, 1 out]
          }
          frame Default {
          }
        }
      }
      frame "Exit" {
        # "Flush the Writer Stream to ensure all pending messages are sent to UI Main VI"
        # "Destroy streams on exit"
        # "Put FPGA VI in a Safe State on Exit"
        # "Stop Message Handling Loop"
        # "Stop All Parallel Loops"
        # "Release the message queue reference"
        # "Exit"
        n99 = call "Enqueue Message.vi"("Message"=w306, "Message Queue"=w305) -> ()  [unwired: 8 in, 2 out]
        n100 = call "Enqueue Message.vi"("Message"=w306, "Message Queue"=w308) -> ()  [unwired: 8 in, 2 out]
        n101 = call "Enqueue Message.vi"("Message"=w306, "Message Queue"=w307) -> ()  [unwired: 8 in, 2 out]
        n102 = call "Enqueue Message.vi"("Message"=w306, "Message Queue"=w309) -> ()  [unwired: 8 in, 2 out]
        n103 = Release Queue(queue=w323, error in (no error)=w319) -> (error out=w321:errorcluster)  [unwired: 1 in, 2 out]
        n104 = global read "Global - RT Stream Connections.vi" "RT Writer Stream"() -> (w312:refnum<k21>)
        n105 = global read "Global - RT Stream Connections.vi" "UI Writer Stream"() -> (w314:refnum<k21>)
        n106 = xnode "Read/Write Control"("FPGA VI Reference In"=w315, "New State"=FPGA_State."Safe State", "Change State"=TRUE) -> ()  [unwired: 1 in, 2 out]
        n107 = Flush Stream(11:w312) -> (0:w310:errorcluster, 3:w311:refnum<k21>)  [unwired: 3 in, 1 out]
        n108 = global write "Global - All RT Loop Stop.vi" "All RT Loop Stop"(TRUE ("Stop Monitoring Loops")) -> ()
        n109 = Destroy Stream Endpoint(8:w310, 11:w311) -> (0:w313:errorcluster)
        n110 = Destroy Stream Endpoint(8:w313, 11:w314) -> ()  [unwired: 1 out]
        n111 = Merge Errors(w321) -> (w320:errorcluster)
      }
      frame "---Copy This Frame---" {
        # "Duplicate this frame when creating new messages.  Change this comment in the duplicated frame to describe this message."
        n112 = Merge Errors(w325) -> (w324:errorcluster)
      }
      frame "Abort" {
        # "Duplicate this frame when creating new messages.  Change this comment in the duplicated frame to describe this message."
        n113 = call "Enqueue Message.vi"("Priority Message? (F)"=TRUE, "Message"="Abort", "Message Queue"=w328) -> ()  [unwired: 7 in, 2 out]
        n114 = flat-sequence {
          frame #0 {
            n115 = global write "Global - Monitoring Variables.vi" "Emergency STOP"(TRUE ("Emergency STOP")) -> ()
          }
          frame #1 {
            n116 = Wait (ms)(milliseconds to wait=u32 500) -> ()  [unwired: 1 out]
          }
          frame #2 {
            n117 = global write "Global - Monitoring Variables.vi" "Emergency STOP"(FALSE ("Emergency STOP")) -> ()
          }
        }
        n118 = Merge Errors(w330) -> (w329:errorcluster)
      }
      frame Default {
        # "'Default' case only runs if there is a message that isn't defined in any of the other cases.  Output a programming error."
        n119 = Format Into String(format string="The invalid message string \"%s\" was received in the Message Handling Loop." ("Unknown Message Error Text"), w337) -> (resulting string=w334:string)  [unwired: 2 in, 1 out]
        n120 = call <vilib>:"Error Cluster From Error Code.vi"("error message (\"\")"=w334, "error code (0)"=1) -> ("error out"=w335:errorcluster)  [unwired: 7 in]
      }
    }
    n121 = call <vilib>:"Clear Errors.vi"("error in (no error)"=w30) -> ("error out"=w24:errorcluster)  [unwired: 5 in, 1 out]
    n122 = call "RT Error Handler - Message Handler.vi"("error in (no error)"=w30, "Message Queue"=w31) -> ()  [unwired: 9 in, 1 out]
  }
  n123 = call "RT Loop - System Health and FPGA Monitoring 9039.vi"("Expansion Chassis Connected?"=w5, "EXPANSION FPGA VI Reference Out"=w4, "FPGA VI Reference"=w8, "Message Queue"=w9) -> ()  [unwired: 8 in]
  n124 = call "RT Loop - AUTO P&D.vi"("FPGA VI Reference"=w8, "P&D Message Queue"=w2, "RT Main Message Queue"=w9) -> ()  [unwired: 8 in]
  n125 = call "Pressurization PID.vi"("Pressure Message Queue"=w1, "Message Queue 2"=w9, "FPGA VI Reference"=w8) -> ()  [unwired: 8 in]
  n126 = call "RT LNG Decoupler State Machine.vi"("FPGA VI Reference"=w8, "Message Queue"=w14, "RT Main Message Queue"=w9) -> ()  [unwired: 8 in]
  n127 = call "RT LOX Decoupler State Machine.vi"("FPGA VI Reference"=w8, "Message Queue"=w13, "RT Main Message Queue"=w9) -> ()  [unwired: 8 in]
  n128 = global read "Global - Configuration Options.vi" "Debugging"() -> (w18:bool)
  n129 = xnode "Close FPGA VI Reference"("FPGA VI Reference In"=w8, "error in"=w6) -> ("error out"=w7:errorcluster)
  n130 = case shown="True" w18 {
    tunnel: w7 -> [_ _]
    frame False {
      n131 = call <vilib>:"Restart.vi"("Session in"=refnum<k21> "localhost" ("session in")) -> ()  [unwired: 8 in, 3 out]
    }
    frame True {
    }
  }
